vi "DRAW_Mouse_body.vi"(0 "Refnum in":T1 caption="Image ref. in", 1 "Mouse color":u32, 2 "Mouse lineout color":u32, 5 "Mouse position, pix":cluster{"Numeric":dbl, "Numeric":dbl}, 7 "Mouse rotation angle, deg":dbl, 9 "Bright mouse lineout":bool, 11 "Error In (no error)":errorcluster, 12 "Mouse size, pix":dbl, 13 "Eye size factor":dbl, 14 "Iris size factor":dbl) -> (4 "Image ref. out":T1, 15 "Error Out":errorcluster)   [LabVIEW 2018, in "Tracker.lvlib"]
uses:
  Tracker.lvlib
  <vilib>/vision/Image Controls.llb/IMAQ Image.ctl
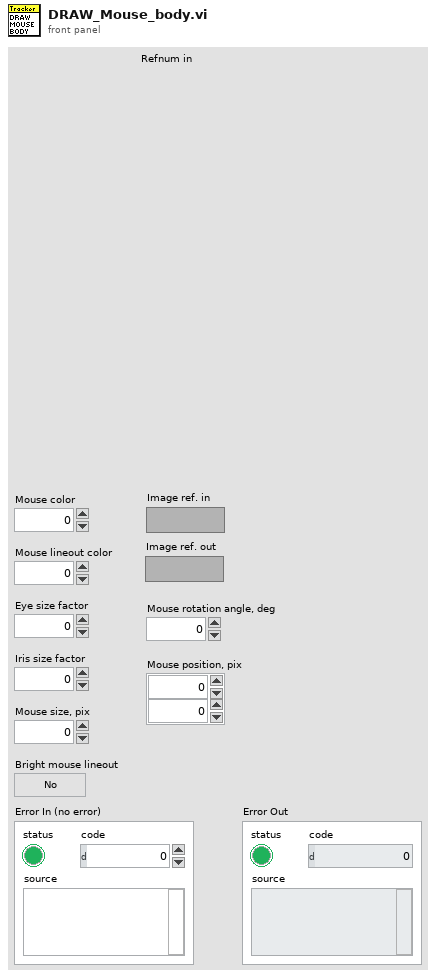
[diagram p1: front panel]
types:
  T1 = typedef "IMAQ Image.ctl" = refnum<image>
  T2 = cluster{"Top":i32, "Left":i32, "Bottom":i32, "Right":i32}
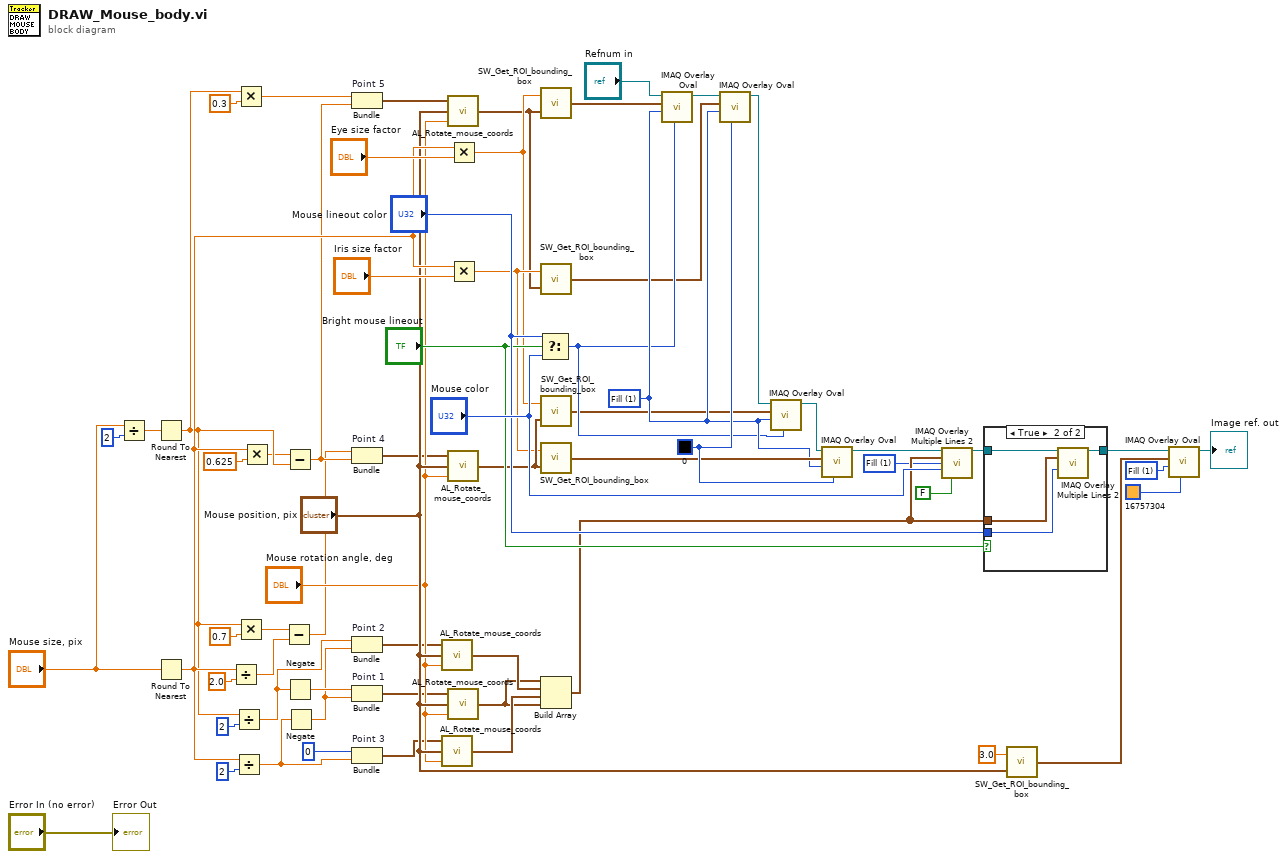
[diagram p0: block diagram]
diagram:
  w52 = u32 0 ("Color")
  w48 = u32 1 items=["Frame", "Fill"] ("Drawing Mode (Frame)")
  w35 = u32 1 items=["Frame", "Fill"] ("Drawing Mode (Frame)")
  w28 = u32 1 items=["Frame", "Fill"] ("Drawing Mode (Frame)")
  n1 = Divide(x="Mouse size, pix", y=2) -> (x/y=w56:dbl)
  n2 = Round To Nearest(number=w56) -> (nearest integer value=w59:dbl)
  n3 = Round To Nearest(number="Mouse size, pix") -> (nearest integer value=w60:dbl)
  n4 = Divide(x=w60, y=2.0) -> (x/y=w21:dbl)
  n5 = Divide(x=w59, y=u16 2) -> (x/y=w26:dbl)
  n6 = Divide(x=w60, y=u16 2) -> (x/y=w5:dbl)
  n7 = Multiply(x=w59, y=0.3) -> (x*y=w23:dbl)
  n8 = Multiply(x=w59, y=0.7) -> (x*y=w17:dbl)
  n9 = Multiply(x=w60, y=0.625) -> (x*y=w20:dbl)
  n10 = Subtract(x=w17, y=w21) -> (x-y=w18:dbl)
  n11 = Subtract(x=w20, y=w59) -> (x-y=w19:dbl)
  n12 = Negate(x=w26) -> (-x=w27:dbl)
  n13 = Negate(x=w5) -> (-x=w24:dbl)
  n14 = Bundle "Point 5"(w23, w19) -> (w13:cluster{dbl, dbl})  [unwired: 1 in]
  n15 = Bundle "Point 4"(w18, w19) -> (w12:cluster{dbl, dbl})  [unwired: 1 in]
  n16 = Bundle "Point 2"(w26, w24) -> (w10:cluster{dbl, dbl})  [unwired: 1 in]
  n17 = Bundle "Point 1"(w27, w24) -> (w9:cluster{dbl, dbl})  [unwired: 1 in]
  n18 = Bundle "Point 3"(0, w5) -> (w11:cluster{i32, dbl})  [unwired: 1 in]
  n19 = call "AL_Rotate_mouse_coords.vi"("Mouse angle of rotation, deg"="Mouse rotation angle, deg", "Offset"="Mouse position, pix", "Coordinates to rotate"=w10) -> ("Rotated coordinates"=w15:cluster{"X":dbl, "Y":dbl})
  n20 = call "AL_Rotate_mouse_coords.vi"("Mouse angle of rotation, deg"="Mouse rotation angle, deg", "Offset"="Mouse position, pix", "Coordinates to rotate"=w11) -> ("Rotated coordinates"=w16:cluster{"X":dbl, "Y":dbl})
  n21 = call "AL_Rotate_mouse_coords.vi"("Mouse angle of rotation, deg"="Mouse rotation angle, deg", "Offset"="Mouse position, pix", "Coordinates to rotate"=w13) -> ("Rotated coordinates"=w39:cluster{"X":dbl, "Y":dbl})
  n22 = call "AL_Rotate_mouse_coords.vi"("Mouse angle of rotation, deg"="Mouse rotation angle, deg", "Offset"="Mouse position, pix", "Coordinates to rotate"=w12) -> ("Rotated coordinates"=w50:cluster{"X":dbl, "Y":dbl})
  n23 = call "AL_Rotate_mouse_coords.vi"("Mouse angle of rotation, deg"="Mouse rotation angle, deg", "Offset"="Mouse position, pix", "Coordinates to rotate"=w9) -> ("Rotated coordinates"=w14:cluster{"X":dbl, "Y":dbl})
  n24 = Multiply(x=w60, y="Eye size factor") -> (x*y=w42:dbl)
  n25 = Multiply(x=w60, y="Iris size factor") -> (x*y=w49:dbl)
  n26 = Select(t="Mouse lineout color", s="Bright mouse lineout", f="Mouse color") -> (s? t:f=w45:u32)
  n27 = call "SW_Get_ROI_bounding_box.vi"("Center of the ROI"=w39, "Radius of the ROI, pix"=w42) -> ("Bounding box of the ROI, pix"=w38:T2)
  n28 = call "SW_Get_ROI_bounding_box.vi"("Center of the ROI"=w39, "Radius of the ROI, pix"=w49) -> ("Bounding box of the ROI, pix"=w40:T2)
  n29 = call "SW_Get_ROI_bounding_box.vi"("Center of the ROI"=w50, "Radius of the ROI, pix"=w42) -> ("Bounding box of the ROI, pix"=w44:T2)
  n30 = call "SW_Get_ROI_bounding_box.vi"("Center of the ROI"=w50, "Radius of the ROI, pix"=w49) -> ("Bounding box of the ROI, pix"=w51:T2)
  n31 = Build Array(w14, w15, w16, w14) -> (w31:cluster{"X":dbl, "Y":dbl}[])
  n32 = call "IMAQ Overlay Oval"("Color"=w45, "Drawing Mode (Frame)"=w48, "Bounding Rectangle"=w38, "Image"="Refnum in") -> ("Image Out"=w41:T1)  [unwired: 6 in, 1 out]
  n33 = call "IMAQ Overlay Oval"("Color"=w52, "Drawing Mode (Frame)"=w48, "Bounding Rectangle"=w40, "Image"=w41) -> ("Image Out"=w43:T1)  [unwired: 6 in, 1 out]
  n34 = call "IMAQ Overlay Oval"("Color"=w45, "Drawing Mode (Frame)"=w48, "Bounding Rectangle"=w44, "Image"=w43) -> ("Image Out"=w46:T1)  [unwired: 6 in, 1 out]
  n35 = call "IMAQ Overlay Oval"("Color"=w52, "Drawing Mode (Frame)"=w48, "Bounding Rectangle"=w51, "Image"=w46) -> ("Image Out"=w47:T1)  [unwired: 6 in, 1 out]
  n36 = call "IMAQ Overlay Multiple Lines 2"("Image"=w47, "Line End Points"=w31, "Drawing Mode (Frame)"=w28, "Color"="Mouse color", "Maintain Width?"=FALSE) -> ("Image Out"=w30:T1)  [unwired: 9 in, 1 out]
  n37 = case shown="True" "Bright mouse lineout" {
    tunnel: w30 -> [w65 w69]
    tunnel: [w65 w68] -> w32
    tunnel: "Mouse lineout color" -> [_ w67]
    tunnel: w31 -> [_ w66]
    frame False {
    }
    frame True {
      n38 = call "IMAQ Overlay Multiple Lines 2"("Image"=w69, "Line End Points"=w66, "Color"=w67) -> ("Image Out"=w68:T1)  [unwired: 11 in, 1 out]
    }
  }
  n39 = call "SW_Get_ROI_bounding_box.vi"("Center of the ROI"="Mouse position, pix", "Radius of the ROI, pix"=3.0) -> ("Bounding box of the ROI, pix"=w37:T2)
  n40 = call "IMAQ Overlay Oval"("Color"=u32 16757304 ("color(black)"), "Drawing Mode (Frame)"=w35, "Bounding Rectangle"=w37, "Image"=w32) -> ("Image Out"=→"Image ref. out":T1)  [unwired: 6 in, 1 out]
  "Error Out" <- "Error In (no error)"
